vi "PCO_GetSensorFormat.vi"(8 "error in (no error)":errorcluster {"code" format="%x"}, 11 "ph":u64) -> (0 "error out":errorcluster {"code" format="%x"}, 1 "wSensor":u16(ring) items=["standard", "extended"], 2 "ErrorMessage":i32 format="%x", 3 "ph out":u64)   [LabVIEW 2019, in "SDK.lvlib" / "ImageSensor.lvlib"]
doc: "<b>Description:</b>\nThis function retrieves the current sensor format. In the format [standard] only effective pixels are readout from the sensor. The readout in the format [extended] is camera dependent. Either a distinct region of the sensor is selected or the full sensor including effective, dark, reference and dummy pixels.\n\n<b>Supported camera type:</b>\nAll cameras\n\n<b>Descriptor dependency:</b>\nNone"
uses:
  ImageSensor.lvlib
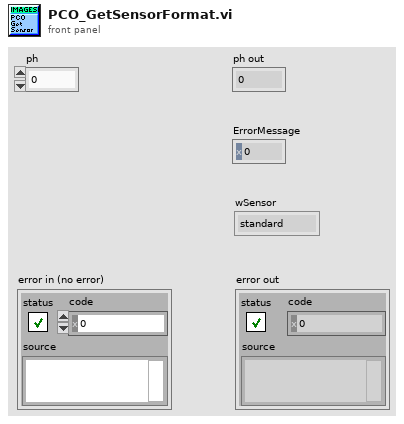
[diagram p1: front panel]
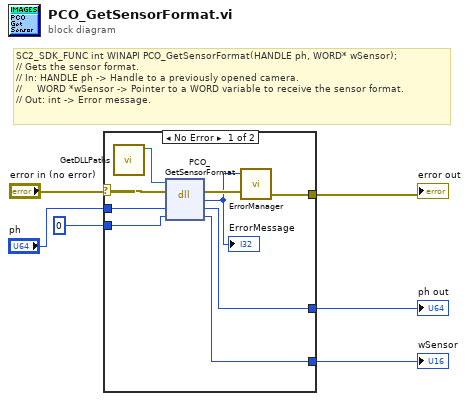
[diagram p0: block diagram]
diagram:
  # "SC2_SDK_FUNC int WINAPI PCO_GetSensorFormat(HANDLE ph, WORD* wSensor);\n// Gets the sensor format.\n// In: HANDLE ph -> Handle to a previously opened camera.\n//     WORD *wSensor -> Pointer to a WORD variable to receive the sensor format.\n// Out: int -> Error message."
  n1 = case shown="No Error" "error in (no error)" {
    selector: "error in (no error)" -> [w8 w18]
    tunnel: "ph" -> [w15 w17]
    tunnel: [w14 w17] -> w5
    tunnel: u16 0 ("wSensor") -> [w13 w16]
    tunnel: [w12 w16] -> w3
    tunnel: [w9 w18] -> w2
    frame No Error {
      n2 = call "GetDLLPaths.vi"() -> ("SC2_Cam_Path"=w7:path)  [unwired: 9 in, 2 out]
      n3 = dll-call lib="?" fn="PCO_GetSensorFormat"(path in=w7, error in=w8, "ph"=w15, "wSensor"=w13) -> (error out=w11:errorcluster, "return type"=w10:i32, "ph"=w14:u64, "wSensor"=w12:u16)  [unwired: 1 in, 1 out]
      "ErrorMessage" <- w10
      n4 = call "ErrorManager.vi"("error in (no error)"=w11, "error code"=w10) -> ("error out"=w9:errorcluster)  [unwired: 3 in]
    }
    frame Error {
    }
  }
  "ph out" <- w5
  "wSensor" <- w3
  "error out" <- w2
